vi "更新显示.vi"(8 "error in (no error)":errorcluster caption="错误输入（无错误）", 11 "生命游戏 输入":refnum<class "生命游戏.lvclass">) -> (0 "error out":errorcluster caption="错误输出", 3 "生命游戏 输出":refnum<class "生命游戏.lvclass">)   [LabVIEW 2015, in "生命游戏.lvlib" / "生命游戏.lvclass"]
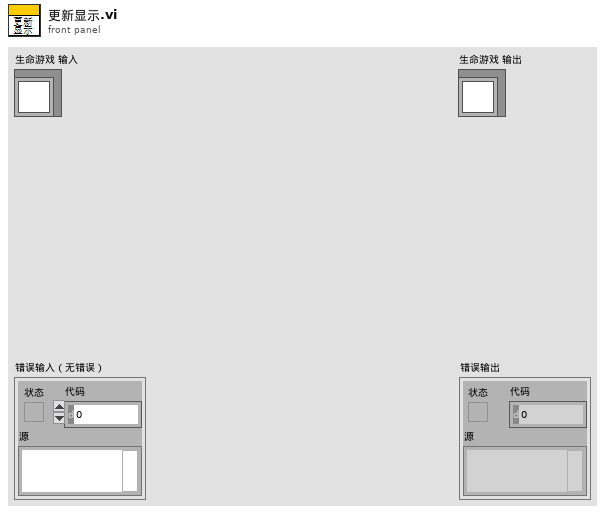
[diagram p1: front panel]
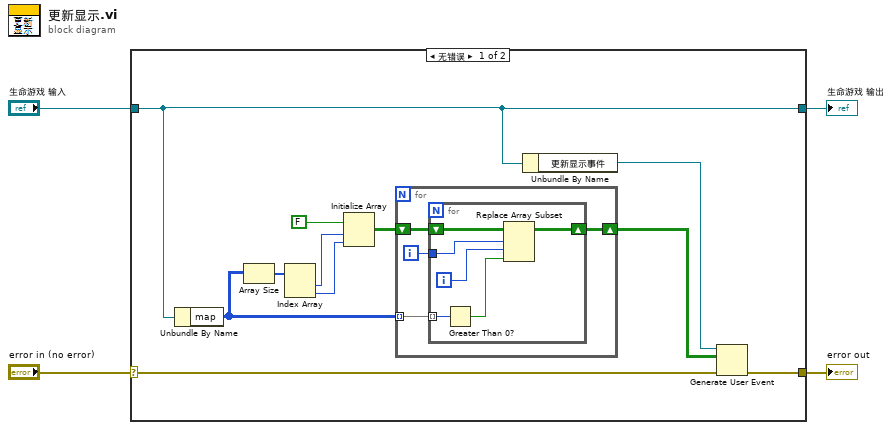
[diagram p0: block diagram]
diagram:
  n1 = case shown="无错误" "error in (no error)" {
    selector: "error in (no error)" -> [w8 w27]
    tunnel: [w7 w27] -> w3
    tunnel: [w9 w26] -> w1
    tunnel: "生命游戏 输入" -> [w9 w26]
    frame No Error {
      n2 = Unbundle By Name(w9) -> ("map"=w10:u8[][])
      n3 = Array Size(array=w10) -> (size(s)=w13:i32[])
      n4 = Index Array(array=w13) -> (element #1=w12:i32, element #2=w11:i32)  [unwired: 2 in]
      n5 = Initialize Array(FALSE, w12, w11) -> (w14:bool[][])
      n6 = for {
        shift-right: [w18] -> w5
        shift-left: w14 -> [w19]
        tunnel: w10 -> [w16] mode=indexing
        i -> [w17]
        n7 = for {
          shift-right: [w24] -> w18
          shift-left: w19 -> [w25]
          tunnel: w17 -> [w23]
          tunnel: w16 -> [w21] mode=indexing
          i -> [w22]
          n8 = Greater Than 0?(x=w21) -> (x > 0?=w20:bool)
          n9 = Replace Array Subset(array=w25, new element=w20, index (row)=w23, index (col)=w22) -> (w24:bool[][])
        }
      }
      n10 = Unbundle By Name(w9) -> ("更新显示事件"=w6:refnum<user-event>)
      n11 = Generate User Event(user event=w6, event data cluster=w5, error in=w8) -> (error out=w7:errorcluster)  [unwired: 1 in, 1 out]
    }
    frame Error {
    }
  }
  "error out" <- w3
  "生命游戏 输出" <- w1
